vi "Header.vi"(0 "Function":string, 2 "Measurement Time":string, 5 "Auto Range":bool=TRUE, 7 "Manual Impedance Range":string, 9 "Signal Frequency":dbl format="%#_13g", 11 "Signal Type":string, 12 "Averaging Factor":i32, 13 "Signal Level":dbl format="%#_13g", 14 "dt":i32) -> (4 "Header":string)   [LabVIEW 2017]
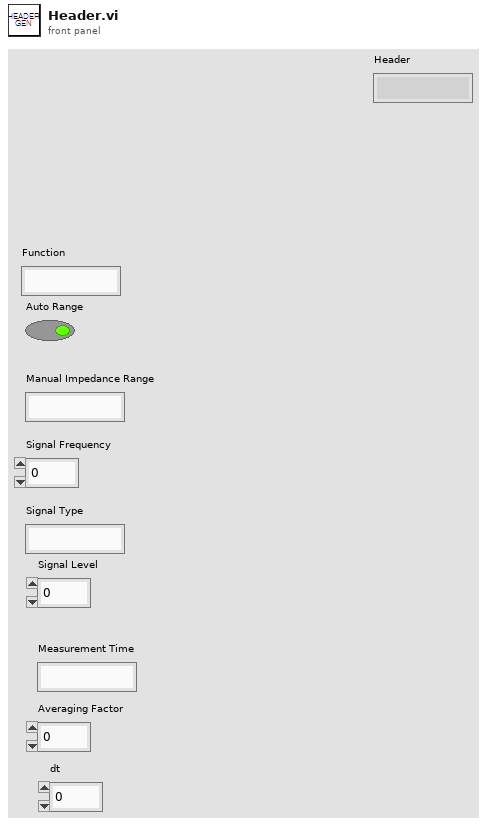
[diagram p1: front panel]
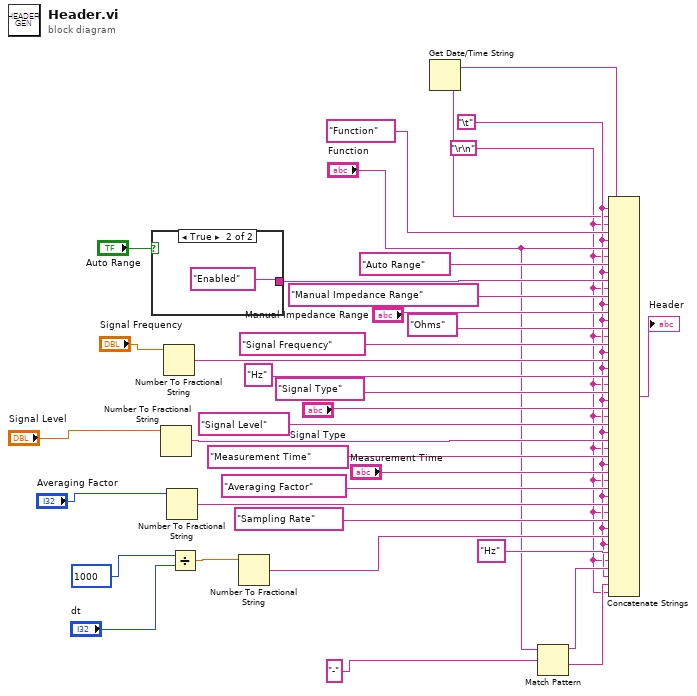
[diagram p0: block diagram]
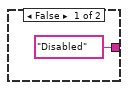
[diagram p2: hidden frame]
diagram:
  w1 = "\r\n"
  w3 = "\t"
  n1 = case shown="True" "Auto Range" {
    tunnel: ["Disabled" "Enabled"] -> w26
    frame False {
    }
    frame True {
    }
  }
  n2 = Number To Fractional String(number="Signal Level") -> (F-format string=w16:string)  [unwired: 3 in]
  n3 = Number To Fractional String(number="Signal Frequency") -> (F-format string=w21:string)  [unwired: 3 in]
  n4 = Number To Fractional String(number="Averaging Factor") -> (F-format string=w12:string)  [unwired: 3 in]
  n5 = Divide(x=1000, y="dt") -> (x/y=w34:dbl)
  n6 = Number To Fractional String(number=w34) -> (F-format string=w10:string)  [unwired: 3 in]
  n7 = Get Date/Time String() -> (date string=w4:string, time string=w2:string)  [unwired: 3 in]
  n8 = Match Pattern(string="Function", regular expression="-") -> (before substring=w6:string, after substring=w5:string)  [unwired: 1 in, 2 out]
  n9 = Concatenate Strings(w4, w3, w2, w1, "Function", w3, "Function", w1, "Auto Range", w3, w26, w1, "Manual Impedance Range", w3, "Manual Impedance Range", w3, "Ohms", w1, "Signal Frequency", w3, w21, w3, "Hz", w1, "Signal Type", w3, "Signal Type", w1, "Signal Level", w3, w16, w1, "Measurement Time", w3, "Measurement Time", w1, "Averaging Factor", w3, w12, w1, "Sampling Rate", w3, w10, w3, "Hz", w1, w6, w3, w5, w1) -> (→"Header":string)
